vi "Renishaw-XL80_GetMeasurementMode.vi"(8 "error in (no error)":errorcluster, 11 "Renishaw-XL80 in":refnum<class "Renishaw-XL80.lvclass">) -> (0 "error out":errorcluster, 2 "MeasurementMode":i32(ring) items=["MEASUREMENT_INDETERMINATE", "MEASUREMENT_LINEAR_PLANE", "MEASUREMENT_LINEAR_RETRO", "MEASUREMENT_ANGULAR", "MEASUREMENT_STRAIGHTNESS_SHORT", "MEASUREMENT_STRAIGHTNESS_LONG", "MEASUREMENT_VELOCITY_RETRO"], 3 "Renishaw-XL80 out":refnum<class "Renishaw-XL80.lvclass">)   [LabVIEW 2024, in "Renishaw-XL80.lvclass"]
doc: "Reading this property retrieves the current measurement mode.\n\nDefinition\nHRESULTget_MeasurementMode( [out, retval] MEASUREMENT_MODES *pVal);\nParameters\npVal\nA variable that will be set to one of the value in the enumerated type MEASUREMENT_MODES\n\nComments\nReading this property will always retrieve the current measurement mode. This mode is the client's requested mode. It may not correspond to the measurement mode returned in the ML10 status, if for instance the ML10 has stopped responding.\n\nThe property will normally return an HRESULT of S_OK. However, it will return E_POINTER if the client supplies a null pointer for pVal.\nThis enumerated type defines constants that specify the measurement mode.\n\nDefinition\n[v1_enum]typedef enum MEASUREMENT_MODES { MEASUREMENT_INDETERMINATE = 0, MEASUREMENT_LINEAR_PLANE = 1, MEASUREMENT_LINEAR_RETRO = 2, MEASUREMENT_ANGULAR = 3, MEASUREMENT_STRAIGHTNESS_SHORT = 4, MEASUREMENT_STRAIGHTNESS_LONG = 5} MEASUREMENT_MODES;\nComments\nThe v1_enum attribute indicates that the enumerated type will be transmitted as a 32-bit entity.\n\nMEASUREMENT_INDETERMINATE may be returned as part of the ML10 status. This would indicate that the ML10 is not responding. Attempting to use this value to set the measurement mode will fail. \nMEASUREMENT_LINEAR_PLANE indicates that the reading is treated as linear using a plane mirror. \nMEASUREMENT_LINEAR_RETRO indicates that the reading is treated as linear using a retro-reflector. \nMEASUREMENT_ANGULAR indicates that the reading is treated as angular. \nMEASUREMENT_STRAIGHTNESS_SHORT indicates that the reading is treated as straightness using short range optics. \nMEASUREMENT_STRAIGHTNESS_LONG indicates that the reading is treated as straightness using long range optics."
uses:
  Renishaw-XL80.lvclass
  Renishaw-XL80.lvclass/Renishaw-XL80.ctl
  D:/A.C.M/Example CSharp_64/bin/Debug/Interop.DX10SDKADAPTORLib.dll
  Example CSharp_64/bin/Debug/Interop.DX10SDKADAPTORLib.dll
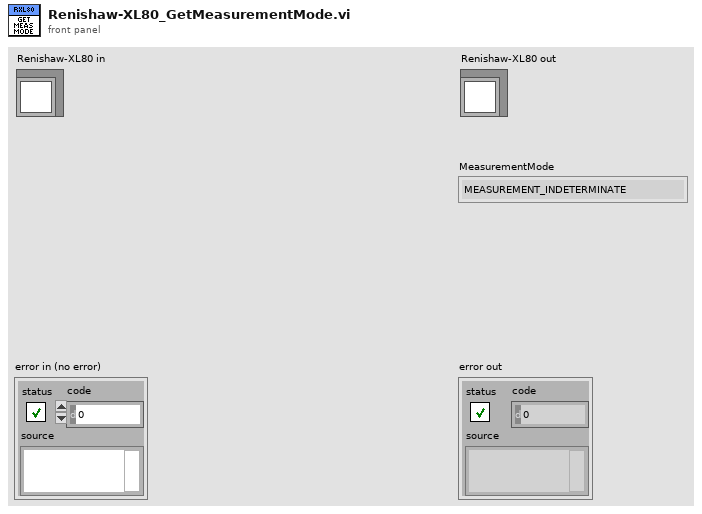
[diagram p1: front panel]
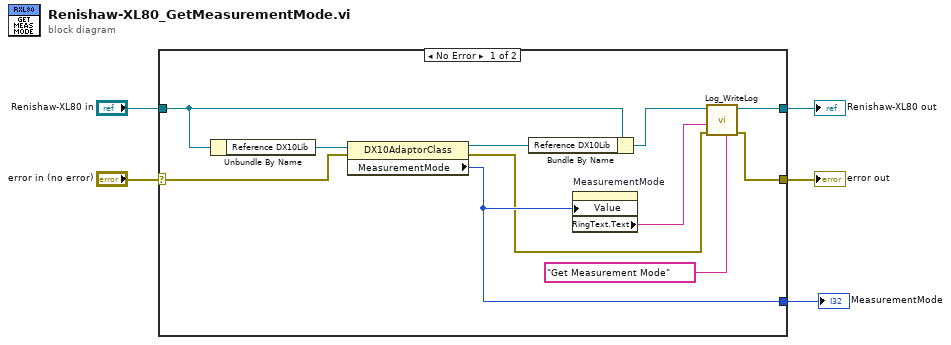
[diagram p0: block diagram]
diagram:
  n1 = case shown="No Error" "error in (no error)" {
    selector: "error in (no error)" -> [w15 w18]
    tunnel: [w7 w18] -> w4
    tunnel: [w12 w17] -> w2
    tunnel: "Renishaw-XL80 in" -> [w14 w17]
    tunnel: [w10 _] -> w1
    frame No Error {
      n2 = Unbundle By Name(w14) -> ("Reference DX10Lib"=w16:refnum<k24>)
      n3 = property class="DX10AdaptorClass"(reference=w16, error in=w15) -> (reference out=w13:refnum<k24>, error out=w6:errorcluster, "MeasurementMode"=w10:i32)
      n4 = Bundle By Name(cluster=w14, "Reference DX10Lib"=w13) -> (w11:refnum<class "Renishaw-XL80.lvclass">)
      n5 = property on="MeasurementMode" class="Ring (strict)"("Value"=w10) -> ("RingText.Text"=w9:string)  [unwired: 2 in, 2 out]
      n6 = call-dynamic "Log_WriteLog.vi"("Additional text"="Get Measurement Mode", "error in (no error)"=w6, "Response"=w9, "Log in"=w11) -> ("error out"=w7:errorcluster, "Log out"=w12:refnum<class "Renishaw-XL80.lvclass">)  [unwired: 6 in]
    }
    frame Error {
    }
  }
  "error out" <- w4
  "Renishaw-XL80 out" <- w2
  "MeasurementMode" <- w1
